vi "JKISM+ TopMain.vi"() -> ()   [LabVIEW 2014]
uses:
  user.lib/_NEVSTOP/JKI State Machine ++/_Support/_JKISMQFGV.vi
  user.lib/_NEVSTOP/JKI State Machine ++/JKI-State-Machine-Plus.lvlib
panel:
  in  "Name(\"\" to use uuid)":string="Event JKISM"
  out "State History":string
  in  "Boolean 2":bool
  in  "Boolean 1":bool
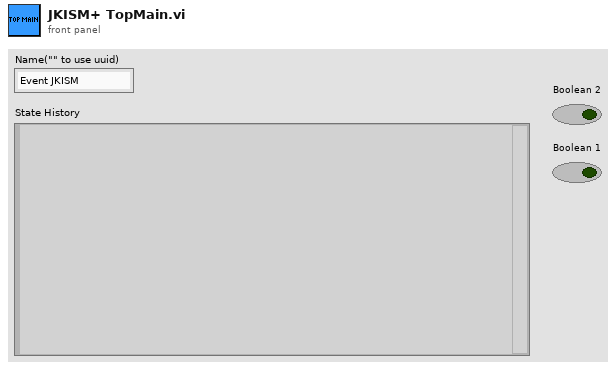
[diagram p1: front panel]
types:
  T1 = enum32{"Invalid", "Standard", "Closed", "Hidden", "Minimized", "Maximized"}
  T2 = enum32{"invalid app kind", "Development System", "Run Time System", "Student Edition", "Embedded LabVIEW", "Evaluation", "Custom"}
  T3 = cluster{"Core":cluster{"Current VI Reference":refnum<vi>, "Close Panel on Exit?":bool}, "Your Boolean data":bool, "Your string data":string}
  T4 = cluster{"Current VI Reference":refnum<vi>, "Close Panel on Exit?":bool}
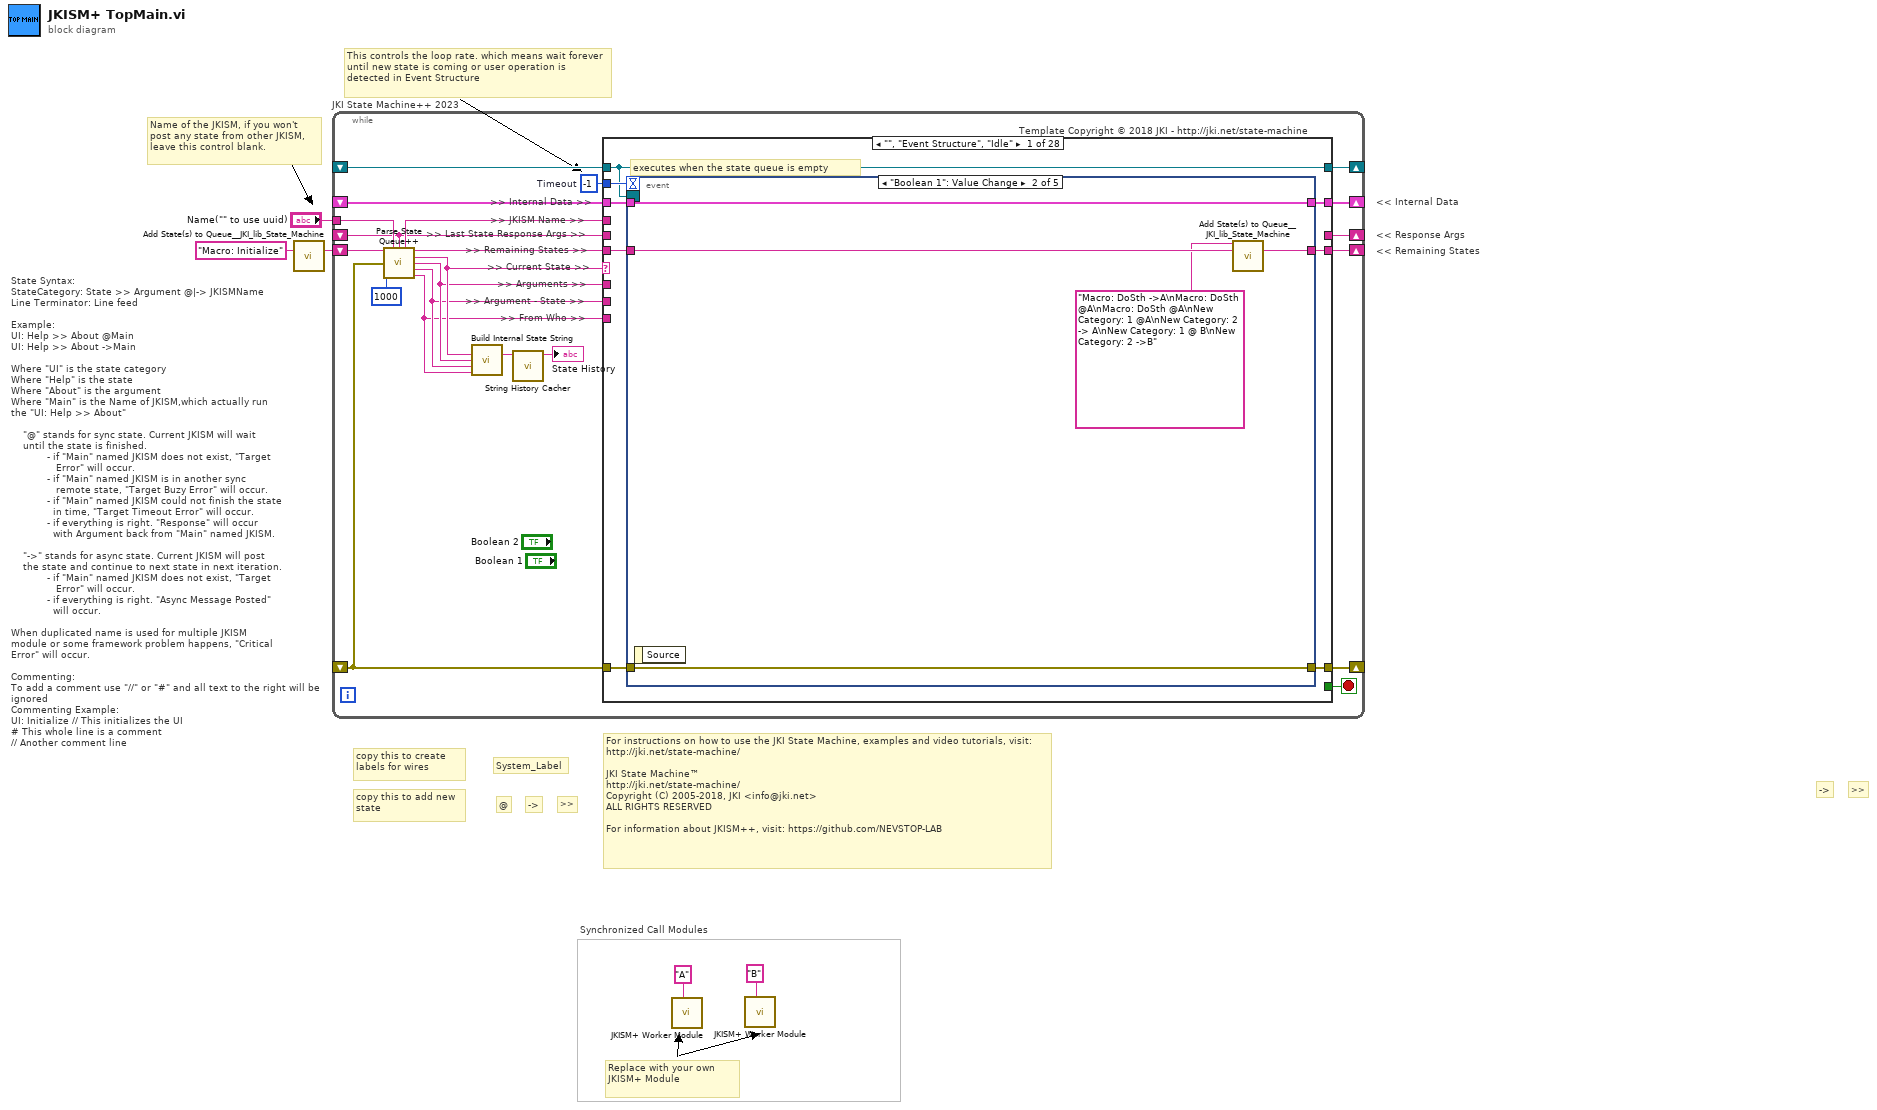
[diagram p0: block diagram]
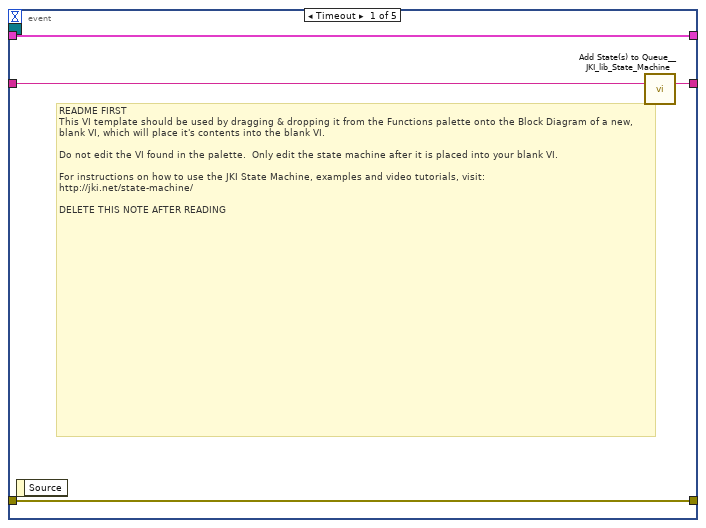
[diagram p2: hidden frame]
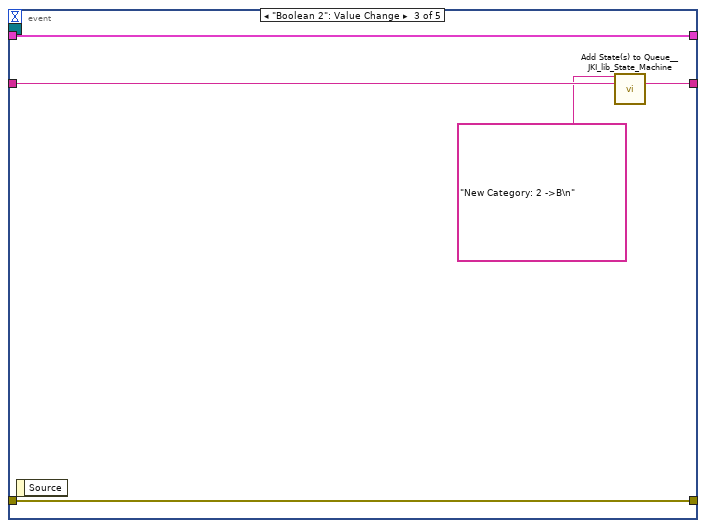
[diagram p3: hidden frame]
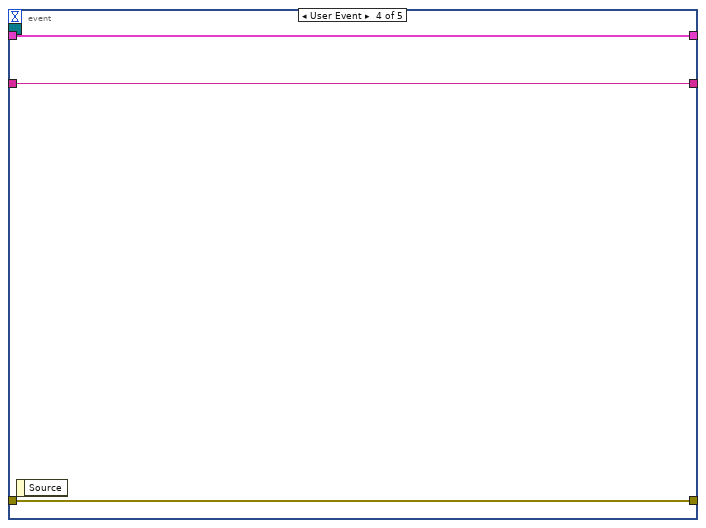
[diagram p4: hidden frame]
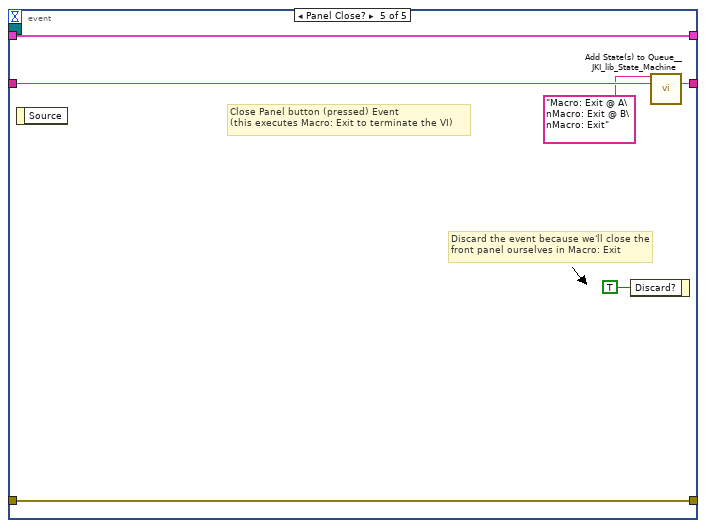
[diagram p5: hidden frame]
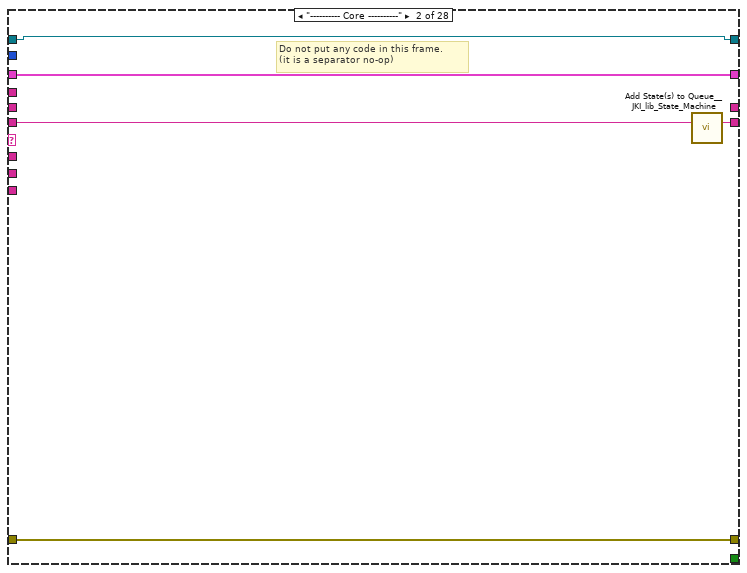
[diagram p6: hidden frame]
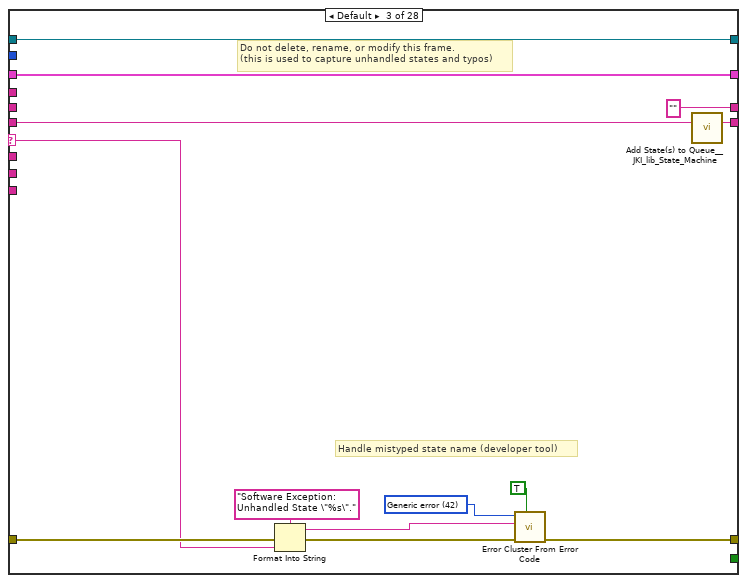
[diagram p7: hidden frame]
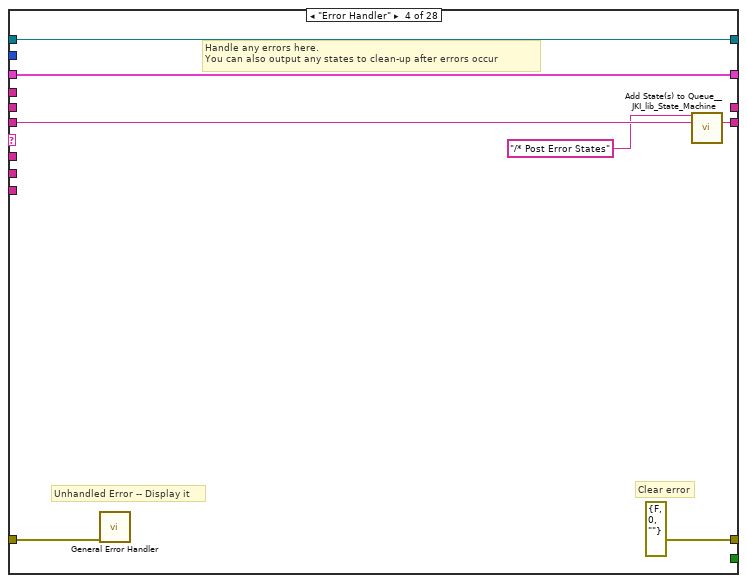
[diagram p8: hidden frame]
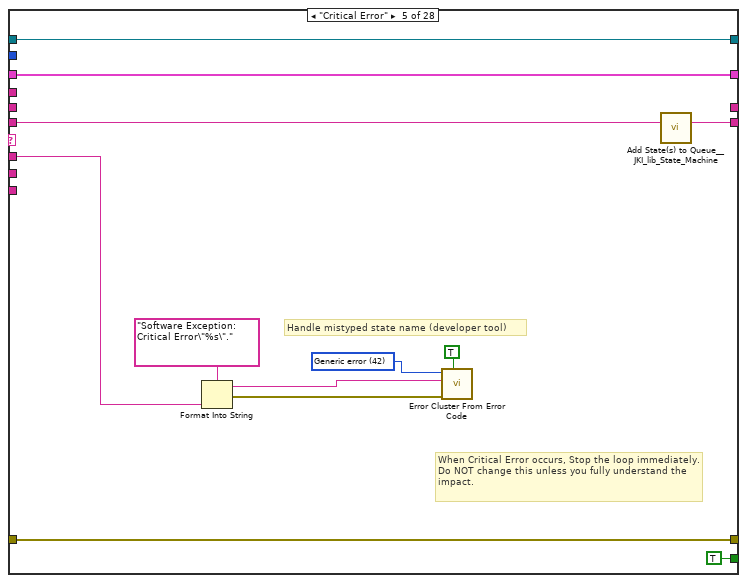
[diagram p9: hidden frame]
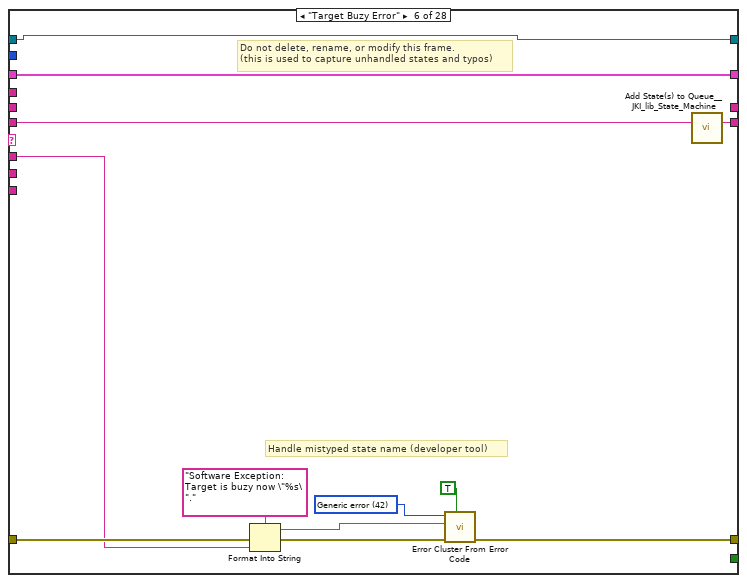
[diagram p10: hidden frame]
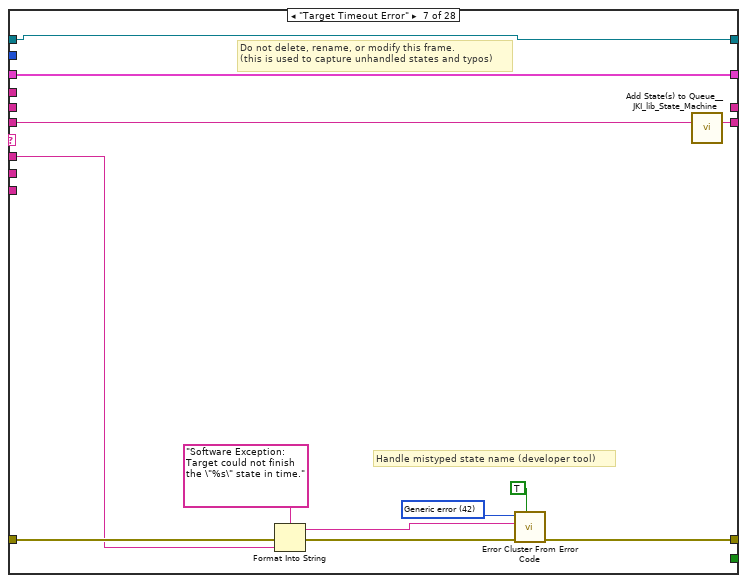
[diagram p11: hidden frame]
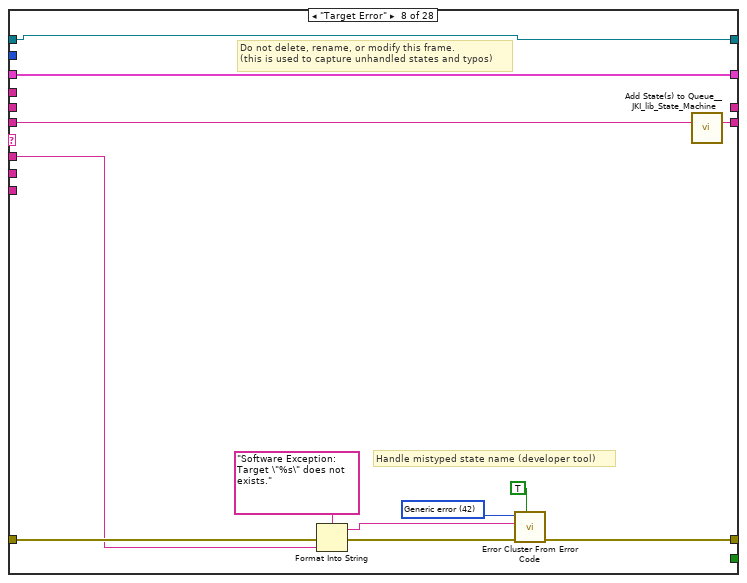
[diagram p12: hidden frame]
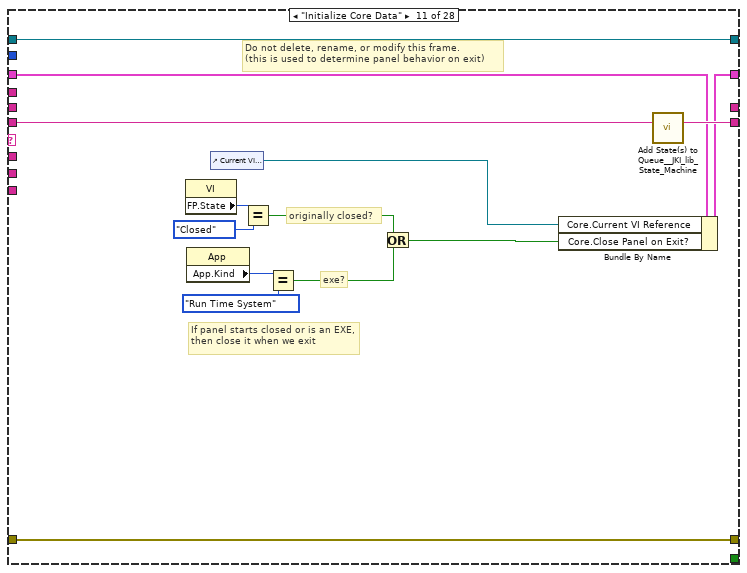
[diagram p15: hidden frame]
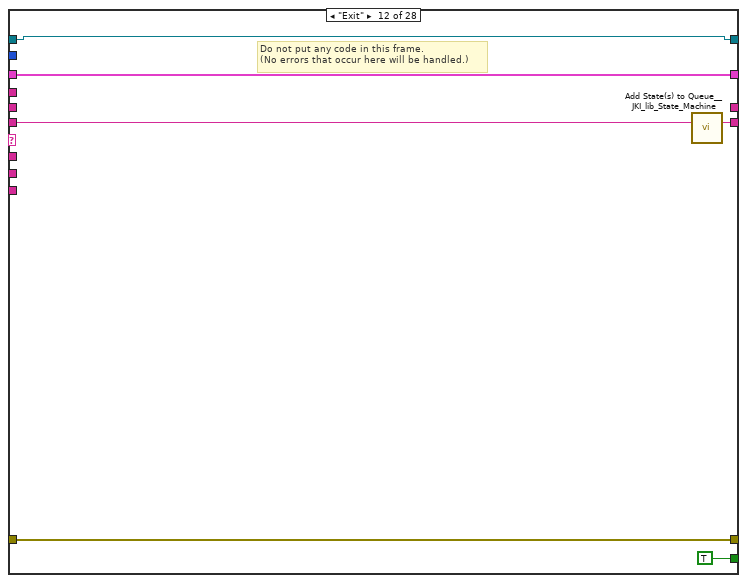
[diagram p16: hidden frame]
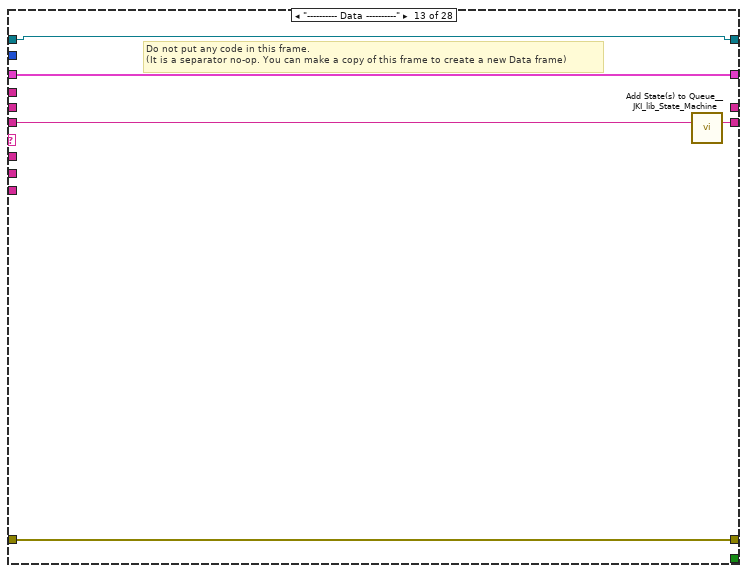
[diagram p17: hidden frame]
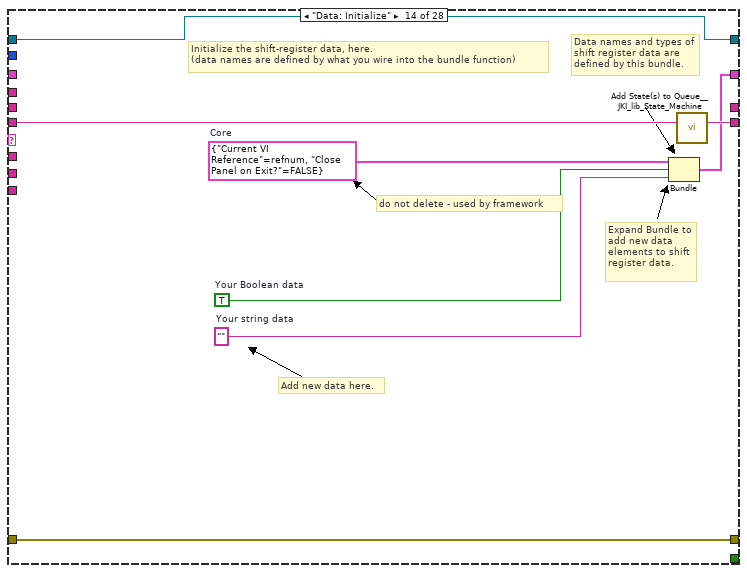
[diagram p18: hidden frame]
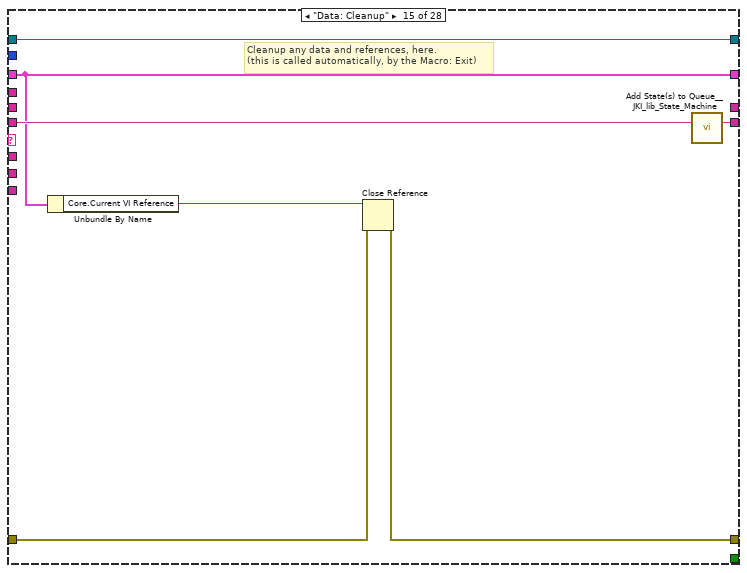
[diagram p19: hidden frame]
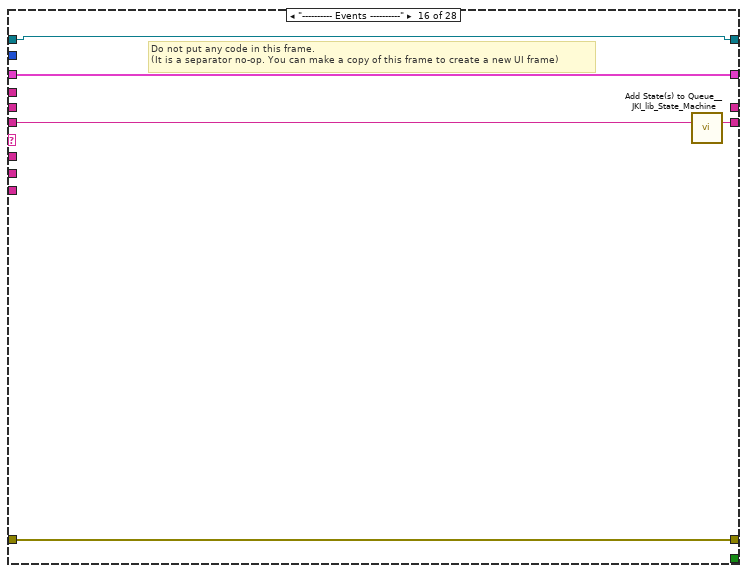
[diagram p20: hidden frame]
diagram:
  # "For instructions on how to use the JKI State Machine, examples and video tutorials, visit: http://jki.net/state-machine/\n\nJKI State Machine™\nhttp://jki.net/state-machine/\nCopyright (C) 2005-2018, JKI <info@jki.net>\nALL RIGHTS RESERVED\n\nFor information about JKISM++, visit: https://github.com/NEVSTOP-LAB"
  # "copy this to add new state"
  # ">>"
  # "->"
  # "@"
  # "State Syntax:\nStateCategory: State >> Argument @|-> JKISMName\nLine Terminator: Line feed\n\nExample:\nUI: Help >> About @Main\nUI: Help >> About ->Main\n\nWhere \"UI\" is the state category\nWhere \"Help\" is the state\nWhere \"About\" is the argument\nWhere \"Main\" is the Name of JKISM,which actually run \nthe \"UI: Help >> About\"\n\n    \"@\" stands for sync state. Current JKISM will wait \n    until the state is finished. \n            - if \"Main\" named JKISM does not exist, \"Target \n               Error\" will occur.\n            - if \"Main\" named JKISM is in another sync \n               remote state, \"Target Buzy Error\" will occur.\n            - if \"Main\" named JKISM could not finish the state \n              in time, \"Target Timeout Error\" will occur.\n            - if everything is right. \"Response\" will occur \n              with Argument back from \"Main\" named JKISM. \n\n    \"->\" stands for async state. Current JKISM will post \n    the state and continue to next state in next iteration.\n            - if \"Main\" named JKISM does not exist, \"Target \n               Error\" will occur.\n            - if everything is right. \"Async Message Posted\"\n              will occur.\n\nWhen duplicated name is used for multiple JKISM \nmodule or some framework problem happens, \"Critical \nError\" will occur.\n\nCommenting:\nTo add a comment use \"//\" or \"#\" and all text to the right will be ignored\nCommenting Example:\nUI: Initialize // This initializes the UI\n# This whole line is a comment\n// Another comment line"
  # "copy this to create labels for wires"
  # "System_Label"
  # ">>"
  # "->"
  # "<< Internal Data"
  # "<< Response Args"
  # "<< Remaining States"
  # "Name of the JKISM, if you won't post any state from other JKISM,  leave this control blank."
  # "This controls the loop rate. which means wait forever until new state is coming or user operation is detected in Event Structure"
  # "Synchronized Call Modules"
  # "Replace with your own JKISM+ Module"
  n1 = call <vilib>:"Add State(s) to Queue__JKI_lib_State_Machine.vi"("State(s) in (\"\")"="Macro: Initialize") -> ("States Out"=w3:string)  [unwired: 14 in]
  n2 = while "JKI State Machine++ 2023" {
    shift-right: [w22] -> _
    shift-left: _ -> [w21]
    shift-right: [w25] -> _
    shift-left: _ -> [w19]
    shift-right: [w24] -> _
    shift-left: w3 -> [w26]
    tunnel: "Name(\"\" to use uuid)" -> [w14]
    shift-right: [w17] -> _
    shift-left: _ -> [w6]
    shift-right: [w16] -> _
    shift-left: _ -> [w15]
    stop <- w23 stop-if-true
    w20 = -1  # Timeout
    # ">> Internal Data >>"
    # ">> Last State Response Args >>"
    # ">> JKISM Name >>"
    # ">> From Who >>"
    # ">> Argument - State >>"
    # ">> Arguments >>"
    # ">> Current State >>"
    # ">> Remaining States >>"
    # "Template Copyright © 2018 JKI - http://jki.net/state-machine"
    n3 = call "Parse State Queue++.vi"("State Queue"=w26, "Name(\"\" to use uuid)"=w14, "Response Arguments"=w6, "Error In (no error)"=w19, "Response Timeout(5000ms)"=1000 ("Response Timeout(1000ms)")) -> ("Name Used"=w7:string, "Remaining States"=w27:string, "Current State"=w11:string, "Arguments"=w10:string, "Argument - State"=w9:string, "From Who"=w8:string)  [unwired: 5 in]
    n4 = call "Build Internal State String.vi"("State"=w11, "Arguments (\"\")"=w10, "Arg-State (\"\")"=w9, "Source (\"\")"=w8) -> ("State with Arguments"=w12:string)  [unwired: 11 in]
    n5 = call "String History Cacher.vi"("String"=w12) -> ("String Cache"=→"State History":string)  [unwired: 10 in]
    n6 = case shown="\"\", \"Event Structure\", \"Idle\"" w11 {
      selector: w11 -> [_ _ w66 _ _ _ _ _ _ _ _ _ _ _ _ _ _ _ _ _ _ _ _ _ _ _ _ _]
      tunnel: w27 -> [w35 w63 w70 w83 w93 w101 w113 w125 w134 w138 w153 w159 w164 w172 w179 w184 w190 w194 w200 w205 w212 w224 w294 w300 w311 w316 w322 w328]
      tunnel: w10 -> [_ _ _ _ w86 w97 w109 w121 _ _ _ _ _ _ _ _ _ _ _ _ w207 w218 _ _ _ _ _ _]
      tunnel: w21 -> [w33 w60 w68 w80 w94 w99 w111 w123 w133 w137 w146 w157 w161 _ w174 w181 w189 w193 w197 w203 w210 w220 w291 w297 w308 w313 w319 w325]
      tunnel: [w32 w61 w72 errorcluster {"status"=FALSE, "code"=0, "source"=""} ("error out") w95 w103 w115 w127 w135 w139 w150 w156 w162 w169 w175 w182 w185 w192 w198 w202 w208 w221 w292 w298 w309 w314 w320 w326] -> w25
      tunnel: w19 -> [w31 w61 w71 w79 w95 w102 w114 w126 w135 w139 w150 w156 w162 w169 w176 w182 _ w195 w198 w202 w209 w222 w292 w298 w309 w314 w320 w326]
      tunnel: [w34 w62 w69 w82 w92 w100 w112 w124 w134 w138 w152 w158 w163 w171 w178 w183 w190 w194 w199 w204 w211 w223 w293 w299 w310 w315 w321 w327] -> w24
      tunnel: [_ _ _ _ TRUE _ _ _ _ _ _ TRUE _ _ _ _ _ _ _ _ _ _ _ _ _ _ _ _] -> w23
      tunnel: [w30 w60 w68 w80 w94 w99 w111 w123 w133 w137 w151 w157 w161 w170 w174 w181 w189 w193 w197 w203 w210 w220 w291 w297 w308 w313 w319 w325] -> w22
      tunnel: w20 -> [w29 _ _ _ _ _ _ _ _ _ _ _ _ _ _ _ _ _ _ _ _ _ _ _ _ _ _ _]
      tunnel: w8 -> [_ _ _ _ _ _ _ _ _ _ _ _ _ _ _ _ _ _ _ _ _ _ _ _ _ _ _ _]
      tunnel: w9 -> [_ _ _ _ _ _ _ _ _ _ _ _ _ _ _ _ _ _ _ _ _ _ _ _ _ _ _ _]
      tunnel: [_ _ "" _ _ _ _ _ _ _ _ _ _ _ _ _ _ _ _ _ _ _ _ _ _ _ "DoA Finished" "DoB Finished"] -> w17
      tunnel: [w28 w59 w64 w77 w84 w96 w108 w120 w132 w136 w140 w154 w160 w165 w173 w180 w188 w191 w196 w201 w206 w217 w290 w295 w301 w312 w318 w324] -> w16
      tunnel: w15 -> [w28 w59 w64 w77 w84 w96 w108 w120 w132 w136 w140 w154 w160 w165 w173 w180 _ w191 w196 w201 w206 w217 w290 w295 w301 w312 w318 w324]
      tunnel: w7 -> [_ _ _ _ _ _ _ _ _ _ _ _ _ _ _ _ w187 _ _ _ _ _ _ _ _ _ _ _]
      tunnel: w6 -> [_ _ _ _ _ _ _ _ _ _ _ _ _ _ _ _ _ _ _ _ _ _ _ _ _ _ _ _]
      frame "", "Event Structure", "Idle" {
        # "executes when the state queue is empty"
        n7 = event shown="[1] \"Boolean 1\": Value Change" {
          selector: w28 -> [_ _ _ _ _]
          dyn-events: _ -> [_ _ _ _ _]
          timeout: w29 -> [_ _ _ _ _]
          tunnel: w35 -> [w39 w42 w47 w51 w58]
          tunnel: [w38 w41 w46 w51 w57] -> w34
          tunnel: w33 -> [w36 w43 w48 w52 w55]
          tunnel: [w37 w44 w49 w50 w56] -> w32
          tunnel: w31 -> [w37 w44 w49 w50 w56]
          tunnel: [w36 w43 w48 w52 w55] -> w30
          event Timeout {
            # "README FIRST\nThis VI template should be used by dragging & dropping it from the Functions palette onto the Block Diagram of a new, blank VI, which will place it's contents into the blank VI.\n\nDo not edit the VI found in the palette.  Only edit the state machine after it is placed into your blank VI.\n\nFor instructions on how to use the JKI State Machine, examples and video tutorials, visit:\nhttp://jki.net/state-machine/\n\nDELETE THIS NOTE AFTER READING"
            n8 = event-data() -> ()  [unwired: 1 in, 1 out]
            n9 = call <vilib>:"Add State(s) to Queue__JKI_lib_State_Machine.vi"("State(s) in (\"\")"=w39) -> ("States Out"=w38:string)  [unwired: 14 in]
          }
          event "Boolean 1": Value Change {
            n10 = event-data() -> ()  [unwired: 1 in, 1 out]
            n11 = call <vilib>:"Add State(s) to Queue__JKI_lib_State_Machine.vi"("State(s) in Front (\"\")"="Macro: DoSth ->A\nMacro: DoSth @A\nMacro: DoSth @A\nNew Category: 1 @A\nNew Category: 2 -> A\nNew Category: 1 @ B\nNew Category: 2 ->B" ("State(s) in Front (\"\")"), "State(s) in (\"\")"=w42) -> ("States Out"=w41:string)  [unwired: 13 in]
          }
          event "Boolean 2": Value Change {
            n12 = event-data() -> ()  [unwired: 1 in, 1 out]
            n13 = call <vilib>:"Add State(s) to Queue__JKI_lib_State_Machine.vi"("State(s) in Front (\"\")"="New Category: 2 ->B\n" ("State(s) in Front (\"\")"), "State(s) in (\"\")"=w47) -> ("States Out"=w46:string)  [unwired: 13 in]
          }
          event User Event {
            n14 = event-data() -> ()  [unwired: 1 in, 1 out]
          }
          event Panel Close? {
            # "Discard the event because we'll close the front panel ourselves in Macro: Exit"
            # "Close Panel button (pressed) Event\n(this executes Macro: Exit to terminate the VI)"
            n15 = event-data() -> ()  [unwired: 1 in, 1 out]
            n16 = event-data("Discard?"=TRUE) -> ()  [unwired: 1 in, 1 out]
            n17 = call <vilib>:"Add State(s) to Queue__JKI_lib_State_Machine.vi"("State(s) in Front (\"\")"="Macro: Exit @ A\nMacro: Exit @ B\nMacro: Exit", "State(s) in (\"\")"=w58) -> ("States Out"=w57:string)  [unwired: 13 in]
          }
        }
      }
      frame "---------- Core ----------" {
        # "Do not put any code in this frame.\n(it is a separator no-op)"
        n18 = call <vilib>:"Add State(s) to Queue__JKI_lib_State_Machine.vi"("State(s) in (\"\")"=w63) -> ("States Out"=w62:string)  [unwired: 14 in]
      }
      frame Default {
        w75 = 42 items=["No error", "Argument error", "Memory is full", "Out of zone", "End of file", "File already open", "Generic file I/O error", "File not found", "File permission error", "Disk is full", "Duplicate path", "Too many files open", "System feature not enabled", "Resource file not found", "Cannot add resource", "Resource not found", "Image not found", "Image memory error", "Pen does not exist", "Config type invalid", "Config token not found", "Config parse error", "Config memory error", "Bad external code format", "Bad external code offset", "External code not present", "Null window", "Destroy window error", "Null menu", "Print aborted", "Bad print record", "Print driver error", "Windows error during printing", "Memory error during printing", "Print dialog error", "Generic print error", "Invalid device refnum", "Device not found", "Device parameter error", "Device unit error", "Cannot open device", "Device call aborted", "Generic error", "Cancelled by user", "Object ID too low", "Object ID too high", "Object not in heap", "Unknown heap", "Unknown object (invalid DefProc)", "Unknown object (DefProc not in table)", "Message out of range", "Invalid (null) method", "Unknown message", "Manager call not supported", "Bad address", "Network operation in progress", "Network operation timed out", "Connection is busy", "Network attribute not supported", "Network error", "Address in use", "System out of memory", "Connection aborted", "Connection refused", "Not connected", "Already connected", "Connection closed", "Initialization error (interapplication manager)", "Bad occurrence", "Wait on unbound occurrence handler", "Occurrence queue overflow", "Datalog type conflict", "Unused", "Unrecognized type (interapplication manager)", "Memory corrupt", "Failed to make temporary DLL", "Old CIN version", "Drag socket not found", "Failed to load drop-object", "Failed to register OLE object", "Failed to release OLE object", "Format specifier type mismatch", "Unknown format specifier", "Too few format specifiers", "Too many format specifiers", "Scan failed", "Newer CIN version", "Error converting to variant", "Runtime menu error", "Password tampered", "Variant attribute not found", "Incompatible variant data type", "Event data is not available", "Event Store is not present", "Occurrence is not found", "Event Queue is not created", "Event info is not available", "Refnum passed is NULL", "Error retrieving Class GUID", "Error retrieving CoClass GUID", "Error retrieving TypeLib GUID.", "Bad built application magic bytes.", "Specific driver is different from the specific driver associated with the Logical Name.", "There is no session opened to the class driver.", "Max Error", "MAX - Error with config objects", "MAX - Error loading configuration", "MAX - Group not supported"]
        # "Do not delete, rename, or modify this frame.\n(this is used to capture unhandled states and typos)"
        # "Handle mistyped state name (developer tool)"
        n19 = Format Into String(format string="Software Exception: Unhandled State \"%s\"." ("message"), error in=w71, w66) -> (resulting string=w74:string, error out=w73:errorcluster)  [unwired: 1 in]
        n20 = call <vilib>:"Error Cluster From Error Code.vi"("show call chain? (False)"=TRUE, "error in (no error)"=w73, "error message (\"\")"=w74, "error code (0)"=w75) -> ("error out"=w72:errorcluster)  [unwired: 5 in]
        n21 = call <vilib>:"Add State(s) to Queue__JKI_lib_State_Machine.vi"("State(s) in (\"\")"=w70) -> ("States Out"=w69:string)  [unwired: 14 in]
      }
      frame "Error Handler" {
        # "Unhandled Error -- Display it"
        # "Handle any errors here.\nYou can also output any states to clean-up after errors occur"
        # "Clear error"
        n22 = call <vilib>:"General Error Handler.vi"("error in (no error)"=w79) -> ()  [unwired: 10 in, 5 out]
        n23 = call <vilib>:"Add State(s) to Queue__JKI_lib_State_Machine.vi"("State(s) in Front (\"\")"="/* Post Error States", "State(s) in (\"\")"=w83) -> ("States Out"=w82:string)  [unwired: 13 in]
      }
      frame "Critical Error" {
        w90 = 42 items=["No error", "Argument error", "Memory is full", "Out of zone", "End of file", "File already open", "Generic file I/O error", "File not found", "File permission error", "Disk is full", "Duplicate path", "Too many files open", "System feature not enabled", "Resource file not found", "Cannot add resource", "Resource not found", "Image not found", "Image memory error", "Pen does not exist", "Config type invalid", "Config token not found", "Config parse error", "Config memory error", "Bad external code format", "Bad external code offset", "External code not present", "Null window", "Destroy window error", "Null menu", "Print aborted", "Bad print record", "Print driver error", "Windows error during printing", "Memory error during printing", "Print dialog error", "Generic print error", "Invalid device refnum", "Device not found", "Device parameter error", "Device unit error", "Cannot open device", "Device call aborted", "Generic error", "Cancelled by user", "Object ID too low", "Object ID too high", "Object not in heap", "Unknown heap", "Unknown object (invalid DefProc)", "Unknown object (DefProc not in table)", "Message out of range", "Invalid (null) method", "Unknown message", "Manager call not supported", "Bad address", "Network operation in progress", "Network operation timed out", "Connection is busy", "Network attribute not supported", "Network error", "Address in use", "System out of memory", "Connection aborted", "Connection refused", "Not connected", "Already connected", "Connection closed", "Initialization error (interapplication manager)", "Bad occurrence", "Wait on unbound occurrence handler", "Occurrence queue overflow", "Datalog type conflict", "Unused", "Unrecognized type (interapplication manager)", "Memory corrupt", "Failed to make temporary DLL", "Old CIN version", "Drag socket not found", "Failed to load drop-object", "Failed to register OLE object", "Failed to release OLE object", "Format specifier type mismatch", "Unknown format specifier", "Too few format specifiers", "Too many format specifiers", "Scan failed", "Newer CIN version", "Error converting to variant", "Runtime menu error", "Password tampered", "Variant attribute not found", "Incompatible variant data type", "Event data is not available", "Event Store is not present", "Occurrence is not found", "Event Queue is not created", "Event info is not available", "Refnum passed is NULL", "Error retrieving Class GUID", "Error retrieving CoClass GUID", "Error retrieving TypeLib GUID.", "Bad built application magic bytes.", "Specific driver is different from the specific driver associated with the Logical Name.", "There is no session opened to the class driver.", "Max Error", "MAX - Error with config objects", "MAX - Error loading configuration", "MAX - Group not supported"]
        # "When Critical Error occurs, Stop the loop immediately. Do NOT change this unless you fully understand the impact."
        # "Handle mistyped state name (developer tool)"
        n24 = Format Into String(format string="Software Exception: Critical Error\"%s\"." ("message"), w86) -> (resulting string=w89:string, error out=w88:errorcluster)  [unwired: 2 in]
        n25 = call <vilib>:"Error Cluster From Error Code.vi"("show call chain? (False)"=TRUE, "error in (no error)"=w88, "error message (\"\")"=w89, "error code (0)"=w90) -> ()  [unwired: 5 in, 1 out]
        n26 = call <vilib>:"Add State(s) to Queue__JKI_lib_State_Machine.vi"("State(s) in (\"\")"=w93) -> ("States Out"=w92:string)  [unwired: 14 in]
      }
      frame "Target Buzy Error" {
        w106 = 42 items=["No error", "Argument error", "Memory is full", "Out of zone", "End of file", "File already open", "Generic file I/O error", "File not found", "File permission error", "Disk is full", "Duplicate path", "Too many files open", "System feature not enabled", "Resource file not found", "Cannot add resource", "Resource not found", "Image not found", "Image memory error", "Pen does not exist", "Config type invalid", "Config token not found", "Config parse error", "Config memory error", "Bad external code format", "Bad external code offset", "External code not present", "Null window", "Destroy window error", "Null menu", "Print aborted", "Bad print record", "Print driver error", "Windows error during printing", "Memory error during printing", "Print dialog error", "Generic print error", "Invalid device refnum", "Device not found", "Device parameter error", "Device unit error", "Cannot open device", "Device call aborted", "Generic error", "Cancelled by user", "Object ID too low", "Object ID too high", "Object not in heap", "Unknown heap", "Unknown object (invalid DefProc)", "Unknown object (DefProc not in table)", "Message out of range", "Invalid (null) method", "Unknown message", "Manager call not supported", "Bad address", "Network operation in progress", "Network operation timed out", "Connection is busy", "Network attribute not supported", "Network error", "Address in use", "System out of memory", "Connection aborted", "Connection refused", "Not connected", "Already connected", "Connection closed", "Initialization error (interapplication manager)", "Bad occurrence", "Wait on unbound occurrence handler", "Occurrence queue overflow", "Datalog type conflict", "Unused", "Unrecognized type (interapplication manager)", "Memory corrupt", "Failed to make temporary DLL", "Old CIN version", "Drag socket not found", "Failed to load drop-object", "Failed to register OLE object", "Failed to release OLE object", "Format specifier type mismatch", "Unknown format specifier", "Too few format specifiers", "Too many format specifiers", "Scan failed", "Newer CIN version", "Error converting to variant", "Runtime menu error", "Password tampered", "Variant attribute not found", "Incompatible variant data type", "Event data is not available", "Event Store is not present", "Occurrence is not found", "Event Queue is not created", "Event info is not available", "Refnum passed is NULL", "Error retrieving Class GUID", "Error retrieving CoClass GUID", "Error retrieving TypeLib GUID.", "Bad built application magic bytes.", "Specific driver is different from the specific driver associated with the Logical Name.", "There is no session opened to the class driver.", "Max Error", "MAX - Error with config objects", "MAX - Error loading configuration", "MAX - Group not supported"]
        # "Do not delete, rename, or modify this frame.\n(this is used to capture unhandled states and typos)"
        # "Handle mistyped state name (developer tool)"
        n27 = Format Into String(format string="Software Exception: Target is buzy now \"%s\"." ("message"), error in=w102, w97) -> (resulting string=w105:string, error out=w104:errorcluster)  [unwired: 1 in]
        n28 = call <vilib>:"Error Cluster From Error Code.vi"("show call chain? (False)"=TRUE, "error in (no error)"=w104, "error message (\"\")"=w105, "error code (0)"=w106) -> ("error out"=w103:errorcluster)  [unwired: 5 in]
        n29 = call <vilib>:"Add State(s) to Queue__JKI_lib_State_Machine.vi"("State(s) in (\"\")"=w101) -> ("States Out"=w100:string)  [unwired: 14 in]
      }
      frame "Target Timeout Error" {
        w118 = 42 items=["No error", "Argument error", "Memory is full", "Out of zone", "End of file", "File already open", "Generic file I/O error", "File not found", "File permission error", "Disk is full", "Duplicate path", "Too many files open", "System feature not enabled", "Resource file not found", "Cannot add resource", "Resource not found", "Image not found", "Image memory error", "Pen does not exist", "Config type invalid", "Config token not found", "Config parse error", "Config memory error", "Bad external code format", "Bad external code offset", "External code not present", "Null window", "Destroy window error", "Null menu", "Print aborted", "Bad print record", "Print driver error", "Windows error during printing", "Memory error during printing", "Print dialog error", "Generic print error", "Invalid device refnum", "Device not found", "Device parameter error", "Device unit error", "Cannot open device", "Device call aborted", "Generic error", "Cancelled by user", "Object ID too low", "Object ID too high", "Object not in heap", "Unknown heap", "Unknown object (invalid DefProc)", "Unknown object (DefProc not in table)", "Message out of range", "Invalid (null) method", "Unknown message", "Manager call not supported", "Bad address", "Network operation in progress", "Network operation timed out", "Connection is busy", "Network attribute not supported", "Network error", "Address in use", "System out of memory", "Connection aborted", "Connection refused", "Not connected", "Already connected", "Connection closed", "Initialization error (interapplication manager)", "Bad occurrence", "Wait on unbound occurrence handler", "Occurrence queue overflow", "Datalog type conflict", "Unused", "Unrecognized type (interapplication manager)", "Memory corrupt", "Failed to make temporary DLL", "Old CIN version", "Drag socket not found", "Failed to load drop-object", "Failed to register OLE object", "Failed to release OLE object", "Format specifier type mismatch", "Unknown format specifier", "Too few format specifiers", "Too many format specifiers", "Scan failed", "Newer CIN version", "Error converting to variant", "Runtime menu error", "Password tampered", "Variant attribute not found", "Incompatible variant data type", "Event data is not available", "Event Store is not present", "Occurrence is not found", "Event Queue is not created", "Event info is not available", "Refnum passed is NULL", "Error retrieving Class GUID", "Error retrieving CoClass GUID", "Error retrieving TypeLib GUID.", "Bad built application magic bytes.", "Specific driver is different from the specific driver associated with the Logical Name.", "There is no session opened to the class driver.", "Max Error", "MAX - Error with config objects", "MAX - Error loading configuration", "MAX - Group not supported"]
        # "Do not delete, rename, or modify this frame.\n(this is used to capture unhandled states and typos)"
        # "Handle mistyped state name (developer tool)"
        n30 = Format Into String(format string="Software Exception: Target could not finish the \"%s\" state in time." ("message"), error in=w114, w109) -> (resulting string=w117:string, error out=w116:errorcluster)  [unwired: 1 in]
        n31 = call <vilib>:"Error Cluster From Error Code.vi"("show call chain? (False)"=TRUE, "error in (no error)"=w116, "error message (\"\")"=w117, "error code (0)"=w118) -> ("error out"=w115:errorcluster)  [unwired: 5 in]
        n32 = call <vilib>:"Add State(s) to Queue__JKI_lib_State_Machine.vi"("State(s) in (\"\")"=w113) -> ("States Out"=w112:string)  [unwired: 14 in]
      }
      frame "Target Error" {
        w130 = 42 items=["No error", "Argument error", "Memory is full", "Out of zone", "End of file", "File already open", "Generic file I/O error", "File not found", "File permission error", "Disk is full", "Duplicate path", "Too many files open", "System feature not enabled", "Resource file not found", "Cannot add resource", "Resource not found", "Image not found", "Image memory error", "Pen does not exist", "Config type invalid", "Config token not found", "Config parse error", "Config memory error", "Bad external code format", "Bad external code offset", "External code not present", "Null window", "Destroy window error", "Null menu", "Print aborted", "Bad print record", "Print driver error", "Windows error during printing", "Memory error during printing", "Print dialog error", "Generic print error", "Invalid device refnum", "Device not found", "Device parameter error", "Device unit error", "Cannot open device", "Device call aborted", "Generic error", "Cancelled by user", "Object ID too low", "Object ID too high", "Object not in heap", "Unknown heap", "Unknown object (invalid DefProc)", "Unknown object (DefProc not in table)", "Message out of range", "Invalid (null) method", "Unknown message", "Manager call not supported", "Bad address", "Network operation in progress", "Network operation timed out", "Connection is busy", "Network attribute not supported", "Network error", "Address in use", "System out of memory", "Connection aborted", "Connection refused", "Not connected", "Already connected", "Connection closed", "Initialization error (interapplication manager)", "Bad occurrence", "Wait on unbound occurrence handler", "Occurrence queue overflow", "Datalog type conflict", "Unused", "Unrecognized type (interapplication manager)", "Memory corrupt", "Failed to make temporary DLL", "Old CIN version", "Drag socket not found", "Failed to load drop-object", "Failed to register OLE object", "Failed to release OLE object", "Format specifier type mismatch", "Unknown format specifier", "Too few format specifiers", "Too many format specifiers", "Scan failed", "Newer CIN version", "Error converting to variant", "Runtime menu error", "Password tampered", "Variant attribute not found", "Incompatible variant data type", "Event data is not available", "Event Store is not present", "Occurrence is not found", "Event Queue is not created", "Event info is not available", "Refnum passed is NULL", "Error retrieving Class GUID", "Error retrieving CoClass GUID", "Error retrieving TypeLib GUID.", "Bad built application magic bytes.", "Specific driver is different from the specific driver associated with the Logical Name.", "There is no session opened to the class driver.", "Max Error", "MAX - Error with config objects", "MAX - Error loading configuration", "MAX - Group not supported"]
        # "Do not delete, rename, or modify this frame.\n(this is used to capture unhandled states and typos)"
        # "Handle mistyped state name (developer tool)"
        n33 = Format Into String(format string="Software Exception: Target \"%s\" does not exists." ("message"), error in=w126, w121) -> (resulting string=w129:string, error out=w128:errorcluster)  [unwired: 1 in]
        n34 = call <vilib>:"Error Cluster From Error Code.vi"("show call chain? (False)"=TRUE, "error in (no error)"=w128, "error message (\"\")"=w129, "error code (0)"=w130) -> ("error out"=w127:errorcluster)  [unwired: 5 in]
        n35 = call <vilib>:"Add State(s) to Queue__JKI_lib_State_Machine.vi"("State(s) in (\"\")"=w125) -> ("States Out"=w124:string)  [unwired: 14 in]
      }
      frame "Async Response", "Response" {
      }
      frame "Async Message Posted" {
      }
      frame "Initialize Core Data" {
        # "Do not delete, rename, or modify this frame.\n(this is used to determine panel behavior on exit)"
        # "originally closed?"
        # "exe?"
        # "If panel starts closed or is an EXE, then close it when we exit"
        n36 = property class="VI"() -> ("FP.State"=w143:T1)  [unwired: 2 in, 2 out]
        n37 = property class="App"() -> ("App.Kind"=w149:T2)  [unwired: 2 in, 2 out]
        n38 = control-ref of="Current VI Reference"() -> (w144:refnum<vi>)
        n39 = Equal?(x=w143, y=T1."Closed" ("Front Panel Window:State")) -> (x = y?=w141:bool)
        n40 = Equal?(x=w149, y=T2."Run Time System" ("Application:Kind")) -> (x = y?=w147:bool)
        n41 = Or(x=w141, y=w147) -> (x .or. y?=w145:bool)
        n42 = Bundle By Name(cluster=w146, "Core.Current VI Reference"=w144, "Core.Close Panel on Exit?"=w145) -> (w151:T3)
        n43 = call <vilib>:"Add State(s) to Queue__JKI_lib_State_Machine.vi"("State(s) in (\"\")"=w153) -> ("States Out"=w152:string)  [unwired: 14 in]
      }
      frame "Exit" {
        # "Do not put any code in this frame.\n(No errors that occur here will be handled.)"
        n44 = call <vilib>:"Add State(s) to Queue__JKI_lib_State_Machine.vi"("State(s) in (\"\")"=w159) -> ("States Out"=w158:string)  [unwired: 14 in]
      }
      frame "---------- Data ----------" {
        # "Do not put any code in this frame.\n(It is a separator no-op. You can make a copy of this frame to create a new Data frame)"
        n45 = call <vilib>:"Add State(s) to Queue__JKI_lib_State_Machine.vi"("State(s) in (\"\")"=w164) -> ("States Out"=w163:string)  [unwired: 14 in]
      }
      frame "Data: Initialize" {
        w166 = T4 {"Current VI Reference"=refnum, "Close Panel on Exit?"=FALSE}  # Core
        w168 = TRUE  # Your Boolean data
        w167 = ""  # Your string data
        # "do not delete - used by framework"
        # "Expand Bundle to add new data elements to shift register data."
        # "Add new data here."
        # "Data names and types of shift register data are defined by this bundle."
        # "Initialize the shift-register data, here.\n(data names are defined by what you wire into the bundle function)"
        n46 = Bundle("Core"=w166, "Your Boolean data"=w168, "Your string data"=w167) -> (w170:T3)  [unwired: 1 in]
        n47 = call <vilib>:"Add State(s) to Queue__JKI_lib_State_Machine.vi"("State(s) in (\"\")"=w172) -> ("States Out"=w171:string)  [unwired: 14 in]
      }
      frame "Data: Cleanup" {
        # "Cleanup any data and references, here.\n(this is called automatically, by the Macro: Exit)"
        n48 = Unbundle By Name(w174) -> ("Core.Current VI Reference"=w177:refnum<vi>)
        n49 = Close Reference(reference=w177, error in (no error)=w176) -> (error out=w175:errorcluster)
        n50 = call <vilib>:"Add State(s) to Queue__JKI_lib_State_Machine.vi"("State(s) in (\"\")"=w179) -> ("States Out"=w178:string)  [unwired: 14 in]
      }
      frame "---------- Events ----------" {
        # "Do not put any code in this frame.\n(It is a separator no-op. You can make a copy of this frame to create a new UI frame)"
        n51 = call <vilib>:"Add State(s) to Queue__JKI_lib_State_Machine.vi"("State(s) in (\"\")"=w184) -> ("States Out"=w183:string)  [unwired: 14 in]
      }
      frame "Events: Register" {
        n52 = call "JKISM++ Get New State Notifier Event.vi"("Name(\"\" to use uuid) in"=w187) -> ("Error out"=w185:errorcluster, "New State Notifier Event"=w186:refnum<user-event>)  [unwired: 9 in]
        n53 = register-events(w186) -> (reference out=w188:refnum<event-registration>)  [unwired: 2 in, 1 out]
      }
      frame "Events: Unregister" {
        n54 = Unregister For Events(event registration refnum=w191, error in=w195) -> (error out=w192:errorcluster)
      }
      frame "---------- UI ----------" {
        # "Do not put any code in this frame.\n(It is a separator no-op. You can make a copy of this frame to create a new UI frame)"
        n55 = call <vilib>:"Add State(s) to Queue__JKI_lib_State_Machine.vi"("State(s) in (\"\")"=w200) -> ("States Out"=w199:string)  [unwired: 14 in]
      }
      frame "UI: Initialize" {
        # "Initialize the User Interface, here.\n(this is called automatically, by the Macro: Init)"
        n56 = call <vilib>:"Add State(s) to Queue__JKI_lib_State_Machine.vi"("State(s) in (\"\")"=w205) -> ("States Out"=w204:string)  [unwired: 14 in]
      }
      frame "UI: Cursor Set" {
        # "Argument"
        # "Set and Unset Cursor Busy.\n(Usage: \"UI: Cursor Set >> Busy|Idle\")"
        n57 = case shown="\"Idle\", Default" w207 {
          tunnel: w209 -> [w214 w216]
          tunnel: [w213 w215] -> w208
          frame "Idle", Default {
            n58 = call <vilib>:"Unset Busy.vi"("error in (no error)"=w214) -> ("error out"=w213:errorcluster)  [unwired: 10 in]
          }
          frame "Busy" {
            n59 = call <vilib>:"Set Busy.vi"("error in (no error)"=w216) -> ("error out"=w215:errorcluster)  [unwired: 9 in, 1 out]
          }
        }
        n60 = call <vilib>:"Add State(s) to Queue__JKI_lib_State_Machine.vi"("State(s) in (\"\")"=w212) -> ("States Out"=w211:string)  [unwired: 14 in]
      }
      frame "UI: Front Panel State" {
        # "Argument"
        # "Set Front Panel Open or Closed\n(Usage: \"UI: Front Panel State >> Open|Close\")"
        n61 = Unbundle By Name(w220) -> ("Core.Current VI Reference"=w219:refnum<vi>)
        n62 = case shown="\"Minimize\", \"Minimized\"" w218 {
          tunnel: w222 -> [w230 w245 w256 w269 w282]
          tunnel: [w232 w246 w258 w271 w284] -> w221
          tunnel: w219 -> [w231 w243 w257 w270 w283]
          frame "Open", "Standard", Default {
            w225 = T1."Standard" ("State")
            n63 = property class="VI"(reference=w231, error in=w230) -> (reference out=w228:refnum<vi>, error out=w229:errorcluster, "FP.State"=w227:T1)
            n64 = Not Equal?(x=w227, y=w225) -> (x != y?=w226:bool)
            n65 = case shown="True" w226 {
              tunnel: [w236 w238] -> w232
              tunnel: w229 -> [w235 w238]
              tunnel: w228 -> [w234 _]
              tunnel: w225 -> [w233 _]
              frame True {
                n66 = invoke class="VI" method="FP.Open"(reference=w234, error in=w235, "Activate"=TRUE, "State"=w233) -> (error out=w236:errorcluster)  [unwired: 1 in, 4 out]
              }
              frame False {
              }
            }
          }
          frame "Close", "Closed" {
            n67 = property class="VI"(reference=w243, error in=w245) -> (reference out=w242:refnum<vi>, error out=w244:errorcluster, "FP.State"=w240:T1)
            n68 = Not Equal?(x=w240, y=T1."Closed" ("Front Panel Window:State")) -> (x != y?=w239:bool)
            n69 = case shown="True" w239 {
              tunnel: [w247 w250] -> w246
              tunnel: w244 -> [w247 w249]
              tunnel: w242 -> [_ w248]
              frame False {
              }
              frame True {
                n70 = invoke class="VI" method="FP.Close"(reference=w248, error in=w249) -> (error out=w250:errorcluster)  [unwired: 1 in, 2 out]
              }
            }
          }
          frame "Hidden", "Hide" {
            w251 = T1."Hidden" ("State")
            n71 = property class="VI"(reference=w257, error in=w256) -> (reference out=w254:refnum<vi>, error out=w255:errorcluster, "FP.State"=w253:T1)
            n72 = Not Equal?(x=w253, y=w251) -> (x != y?=w252:bool)
            n73 = case shown="True" w252 {
              tunnel: [w262 w263] -> w258
              tunnel: w255 -> [w261 w263]
              tunnel: w254 -> [w260 _]
              tunnel: w251 -> [w259 _]
              frame True {
                n74 = invoke class="VI" method="FP.Open"(reference=w260, error in=w261, "State"=w259) -> (error out=w262:errorcluster)  [unwired: 2 in, 4 out]
              }
              frame False {
              }
            }
          }
          frame "Minimize", "Minimized" {
            w264 = T1."Minimized" ("State")
            n75 = property class="VI"(reference=w270, error in=w269) -> (reference out=w267:refnum<vi>, error out=w268:errorcluster, "FP.State"=w266:T1)
            n76 = Not Equal?(x=w266, y=w264) -> (x != y?=w265:bool)
            n77 = case shown="True" w265 {
              tunnel: [w275 w276] -> w271
              tunnel: w268 -> [w274 w276]
              tunnel: w267 -> [w273 _]
              tunnel: w264 -> [w272 _]
              frame True {
                n78 = invoke class="VI" method="FP.Open"(reference=w273, error in=w274, "State"=w272) -> (error out=w275:errorcluster)  [unwired: 2 in, 4 out]
              }
              frame False {
              }
            }
          }
          frame "Maximize", "Maximized" {
            w277 = T1."Maximized" ("State")
            n79 = property class="VI"(reference=w283, error in=w282) -> (reference out=w280:refnum<vi>, error out=w281:errorcluster, "FP.State"=w279:T1)
            n80 = Not Equal?(x=w279, y=w277) -> (x != y?=w278:bool)
            n81 = case shown="True" w278 {
              tunnel: [w288 w289] -> w284
              tunnel: w281 -> [w287 w289]
              tunnel: w280 -> [w286 _]
              tunnel: w277 -> [w285 _]
              frame True {
                n82 = invoke class="VI" method="FP.Open"(reference=w286, error in=w287, "State"=w285) -> (error out=w288:errorcluster)  [unwired: 2 in, 4 out]
              }
              frame False {
              }
            }
          }
        }
        n83 = call <vilib>:"Add State(s) to Queue__JKI_lib_State_Machine.vi"("State(s) in (\"\")"=w224) -> ("States Out"=w223:string)  [unwired: 14 in]
      }
      frame "---------- Macro ----------" {
        # "Do not put any code in this frame.\n(It is a separator no-op. You can make a copy of this frame to create a new Macro frame)"
        n84 = call <vilib>:"Add State(s) to Queue__JKI_lib_State_Machine.vi"("State(s) in (\"\")"=w294) -> ("States Out"=w293:string)  [unwired: 14 in]
      }
      frame "Macro: Initialize" {
        w296 = "Data: Initialize\nInitialize Core Data\nEvents: Register\nUI: Initialize\nUI: Front Panel State >> Open"  # Data: Initialize Initialize Core Data Events: Register UI: Initialize UI: Front Panel State >> Open
        # "Initialization Macro\n(This is called once, when the VI starts)"
        n85 = call <vilib>:"Add State(s) to Queue__JKI_lib_State_Machine.vi"("State(s) in Front (\"\")"=w296, "State(s) in (\"\")"=w300) -> ("States Out"=w299:string)  [unwired: 13 in]
      }
      frame "Macro: Exit" {
        # "Exit Macro\n(This is called once, when the VI exits)"
        n86 = Unbundle By Name(w308) -> ("Core.Close Panel on Exit?"=w307:bool)
        n87 = Select(t="UI: Front Panel State >> Close", s=w307, f="") -> (s? t:f=w304:string)
        n88 = call <vilib>:"Add State(s) to Queue__JKI_lib_State_Machine.vi"("State(s) in (\"\")"=w304, "State(s) at Back (\"\")"="Data: Cleanup\nEvents: Unregister\nExit") -> ("States Out"=w302:string)  [unwired: 13 in]
        n89 = call <vilib>:"Add State(s) to Queue__JKI_lib_State_Machine.vi"("State(s) in Front (\"\")"=w302, "State(s) in (\"\")"=w311) -> ("States Out"=w310:string)  [unwired: 13 in]
      }
      frame "---------- DoSth ----------" {
        # "Template Separator\n(You can make a copy of, or modify, this frame)"
        n90 = call <vilib>:"Add State(s) to Queue__JKI_lib_State_Machine.vi"("State(s) in (\"\")"=w316) -> ("States Out"=w315:string)  [unwired: 14 in]
      }
      frame "DoSth: DoA" {
        # "Your code here.\n(You can make a copy of, or modify, this frame)"
        n91 = call <vilib>:"Add State(s) to Queue__JKI_lib_State_Machine.vi"("State(s) in (\"\")"=w322) -> ("States Out"=w321:string)  [unwired: 14 in]
      }
      frame "DoSth: DoB" {
        # "Your code here.\n(You can make a copy of, or modify, this frame)"
        n92 = call <vilib>:"Add State(s) to Queue__JKI_lib_State_Machine.vi"("State(s) in (\"\")"=w328) -> ("States Out"=w327:string)  [unwired: 14 in]
      }
    }
  }
  n93 = call "JKISM+ Worker Module.vi"("Name(\"\" to use uuid)"="A" ("Name")) -> ()  [unwired: 11 in]
  n94 = call "JKISM+ Worker Module.vi"("Name(\"\" to use uuid)"="B" ("Name")) -> ()  [unwired: 11 in]
